vi "Get Data Bit.vi"(8 "error in (no error)":errorcluster caption="entrée d'erreur (pas d'erreur)", 11 "Class UART (Default) en entrée":refnum<class "Class UART (Default).lvclass">) -> (0 "error out":errorcluster caption="sortie d'erreur", 2 "Data Bit":u16, 3 "Class UART (Default) en sortie":refnum<class "Class UART (Default).lvclass">)   [LabVIEW 2020, in "Library Instrument & Equipement.lvlib" / "Library UART.lvlib" / "Class UART (Default).lvclass"]
uses:
  Class UART (Default).lvclass
  Class UART (Default).lvclass/Class UART (Default).ctl
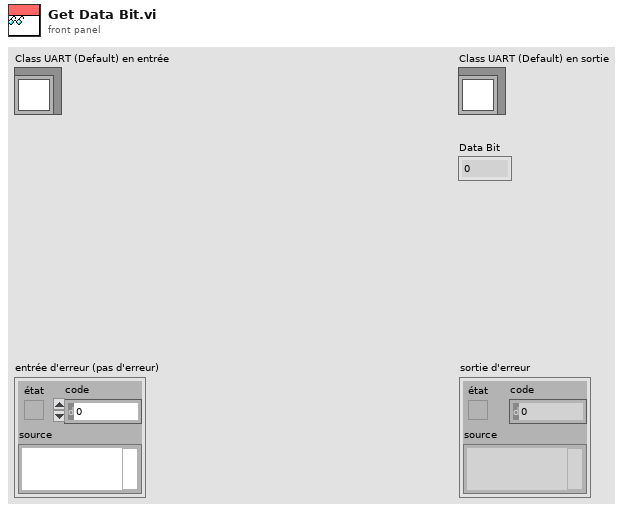
[diagram p1: front panel]
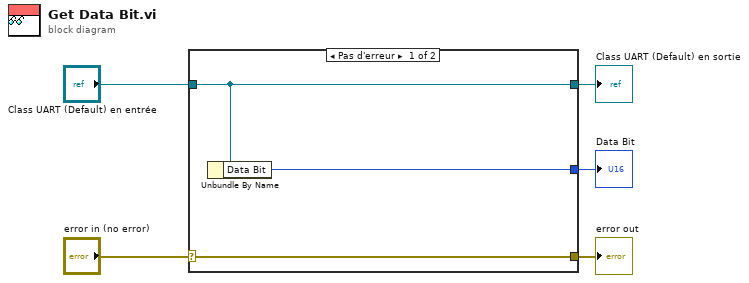
[diagram p0: block diagram]
diagram:
  n1 = case shown="Pas d'erreur" "error in (no error)" {
    selector: "error in (no error)" -> [w8 w9]
    tunnel: [w8 w9] -> w4
    tunnel: [w7 w10] -> w2
    tunnel: "Class UART (Default) en entrée" -> [w7 w10]
    tunnel: [w6 _] -> w1
    frame No Error {
      n2 = Unbundle By Name(w7) -> ("Data Bit"=w6:u16)
    }
    frame Error {
    }
  }
  "error out" <- w4
  "Class UART (Default) en sortie" <- w2
  "Data Bit" <- w1
